vi "Stock Manager.vi"(0 "Stock Manager Action":T1, 7 "String to find (ISIN,Label,Symbol)":string, 12 "Currency (Euro)":T2, 13 "Symbol_Suffix (.PA)":string=".PA") -> (4 "Stocks":refnum<class "Stock.lvclass">[](array[class]), 10 "Stocks Found ?":bool, 15 "Stocks Found":refnum<class "Stock.lvclass">[](array[class]))   [LabVIEW 2012]
uses:
  controls/Currencies.ctl
  Stock/Stock.lvclass
  Stock Manager Action.ctl
  Stock/Stock.lvclass/Stock.ctl
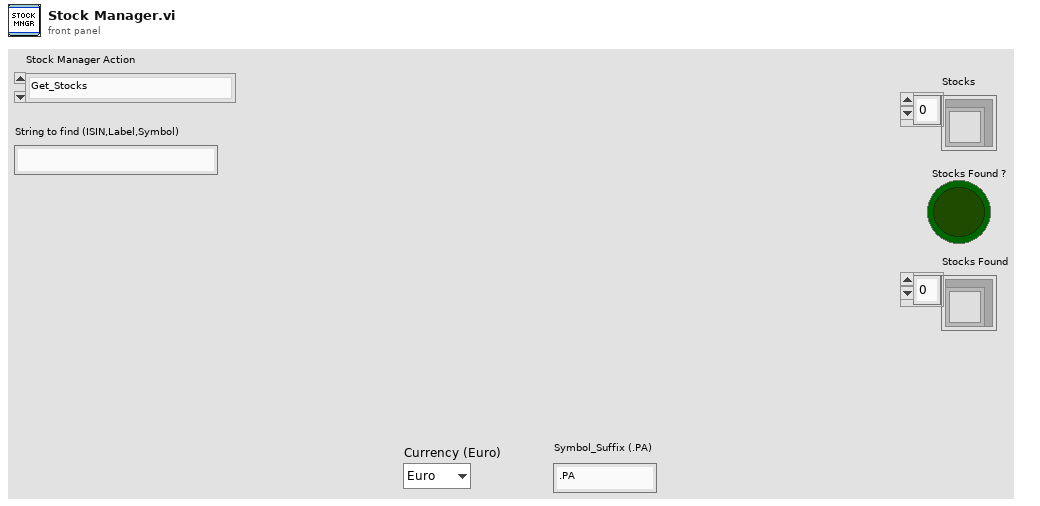
[diagram p1: front panel]
types:
  T1 = typedef "Stock Manager Action.ctl" = enum16{"Get_Stocks", "Load_Stocks", "Find_Stock_From_ISIN", "Find_Stock_From_Label", "Find_Stock_From_Symbol"}
  T2 = typedef "Currencies.ctl" = enum16{"Euro", "Dollar", "Yen", "RIM", "CHF"}
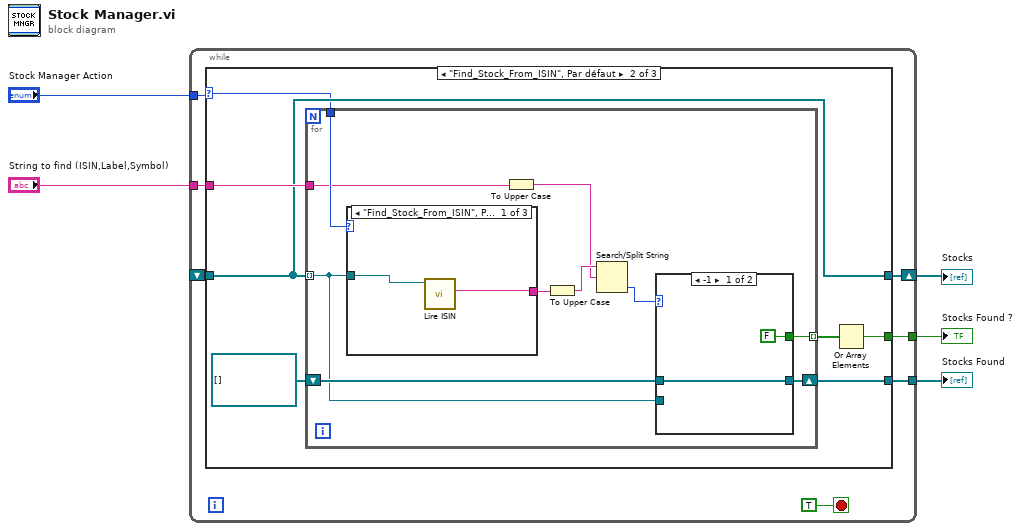
[diagram p0: block diagram]
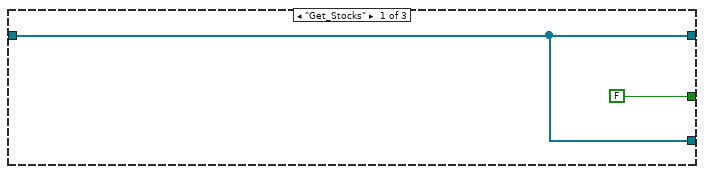
[diagram p2: hidden frame]
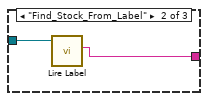
[diagram p3: hidden frame]
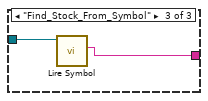
[diagram p4: hidden frame]
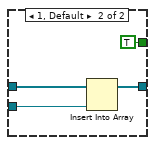
[diagram p5: hidden frame]
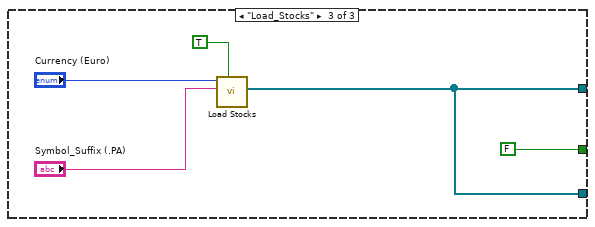
[diagram p6: hidden frame]
diagram:
  n1 = while {
    tunnel: "Stock Manager Action" -> [w11]
    shift-right: [w10] -> w3
    shift-left: _ -> [w9]
    tunnel: "String to find (ISIN,Label,Symbol)" -> [w8]
    tunnel: [w7] -> w2
    tunnel: [w6] -> w1
    stop <- TRUE stop-if-true
    n2 = case shown="\"Find_Stock_From_ISIN\", Par défaut" w11 {
      selector: w11 -> [_ w16 _]
      tunnel: [w13 w20 w44] -> w10
      tunnel: w9 -> [w13 w20 _]
      tunnel: w8 -> [_ w21 _]
      tunnel: [FALSE w18 FALSE] -> w7
      tunnel: [w13 w17 w44] -> w6
      frame "Get_Stocks" {
      }
      frame "Find_Stock_From_ISIN", Default {
        n3 = for {
          tunnel: w20 -> [w28] mode=indexing
          tunnel: w21 -> [w25]
          tunnel: [w31] -> w19 mode=indexing
          shift-right: [w30] -> w17
          shift-left: refnum<class "Stock.lvclass">[] [] -> [w29]
          tunnel: w16 -> [w27]
          n4 = case shown="\"Find_Stock_From_ISIN\", Par défaut" w27 {
            tunnel: [w32 w34 w36] -> w24
            tunnel: w28 -> [w33 w35 w37]
            frame "Find_Stock_From_ISIN", Default {
              n5 = call "Lire ISIN.vi"("Share en entrée"=w33) -> ("ISIN"=w32:string)  [unwired: 8 in, 2 out]
            }
            frame "Find_Stock_From_Label" {
              n6 = call "Lire Label.vi"("Share en entrée"=w35) -> ("Label"=w34:string)  [unwired: 8 in, 2 out]
            }
            frame "Find_Stock_From_Symbol" {
              n7 = call "Lire Symbol.vi"("Share en entrée"=w37) -> ("Symbol"=w36:string)  [unwired: 8 in, 2 out]
            }
          }
          n8 = To Upper Case(1:w25) -> (0:w22:string)
          n9 = To Upper Case(1:w24) -> (0:w23:string)
          n10 = Search/Split String(string=w23, search string/char (-)=w22) -> (offset of match=w26:i32)  [unwired: 1 in, 2 out]
          n11 = case shown="-1" w26 {
            tunnel: w29 -> [w38 w41]
            tunnel: [FALSE TRUE] -> w31
            tunnel: [w38 w42] -> w30
            tunnel: w28 -> [_ w40]
            frame -1 {
            }
            frame 1, Default {
              n12 = Insert Into Array(array=w41, new element=w40) -> (w42:refnum<class "Stock.lvclass">[])  [unwired: 1 in]
            }
          }
        }
        n13 = Or Array Elements(Boolean array=w19) -> (logical OR=w18:bool)
      }
      frame "Load_Stocks" {
        n14 = call "Load Stocks.vi"("Use Default libelle path ? (Y)"=TRUE, "Symbol_Suffix (.PA)"="Symbol_Suffix (.PA)", "Currency (Euro)"="Currency (Euro)") -> ("Stocks"=w44:refnum<class "Stock.lvclass">[])  [unwired: 7 in, 1 out]
      }
    }
  }
  "Stocks" <- w3
  "Stocks Found ?" <- w2
  "Stocks Found" <- w1
